vi "Refresh Param Channels.vi"(8 "error in (no error)":errorcluster, 10 "Label":T1, 11 "Param Ref in":T5 format="%.0x") -> (0 "error out":errorcluster, 3 "Param Ref out":T5 format="%.0x")   [LabVIEW 2015, in "AIT 429 System Explorer.lvlib"]
uses:
  AIT 429 System Explorer.lvlib
  <vilib>/NI Veristand/Custom Device API/Custom Device Item Ref.ctl
  Controls/AIT_Label.ctl
  Controls/AIT_Word.ctl
  Controls/ARINCParam.ctl
  Shared/Controls and Global/TransferType.ctl
  <vilib>/NI Veristand/Custom Device API/Custom Device Channel Type.ctl
  Shared/Controls and Global/Global.vi
  <vilib>/NI Veristand/Custom Device API/Set Item Property (Variant).vi
  <vilib>/NI Veristand/Custom Device Tools/Custom Device Utility Library/NI VeriStand - Search for All Items by GUID.vi
  Shared/AIT 429 Shared.lvlib
  <vilib>/NI Veristand/Custom Device Tools/Custom Device Utility Library/Custom Device Utility Library.lvlib
  <vilib>/NI Veristand/Custom Device API/Custom Device API.lvlib
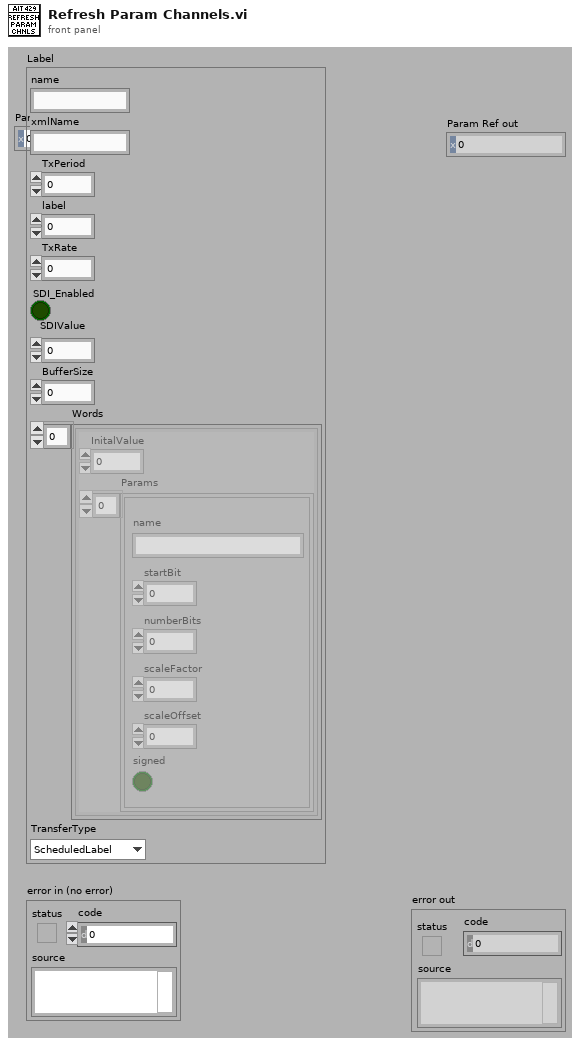
[diagram p1: front panel]
types:
  T1 = typedef "AIT 429 System Explorer.lvlib/AIT_Label.ctl" = cluster{"name":string, "xmlName":string, "TxPeriod":u32, "label":u32, "TxRate":dbl, "SDI_Enabled":bool, "SDIValue":u8, "BufferSize":u32, "Words":T2[], "TransferType":T4}
  T2 = typedef "AIT 429 System Explorer.lvlib/AIT_Word.ctl" = cluster{"InitalValue":u32, "Params":T3[]}
  T3 = typedef "AIT 429 System Explorer.lvlib/ARINCParam.ctl" = cluster{"name":string, "startBit":i32, "numberBits":i32, "scaleFactor":dbl, "scaleOffset":dbl, "signed":bool}
  T4 = typedef "AIT 429 Shared.lvlib/TransferType.ctl" = enum16{"ScheduledLabel", "Acyclic", "Block", "Strobe"}
  T5 = typedef "Custom Device API.lvlib/Custom Device Item Ref.ctl" = u64
  T6 = typedef "Custom Device API.lvlib/Custom Device Channel Type.ctl" = enum16{"Input", "Output"}
  T7 = typedef "Custom Device API.lvlib/Custom Device Item Info.ctl" = cluster{"Name":string, "Is Channel":bool, "GUID":string, "Is Waveform":bool}
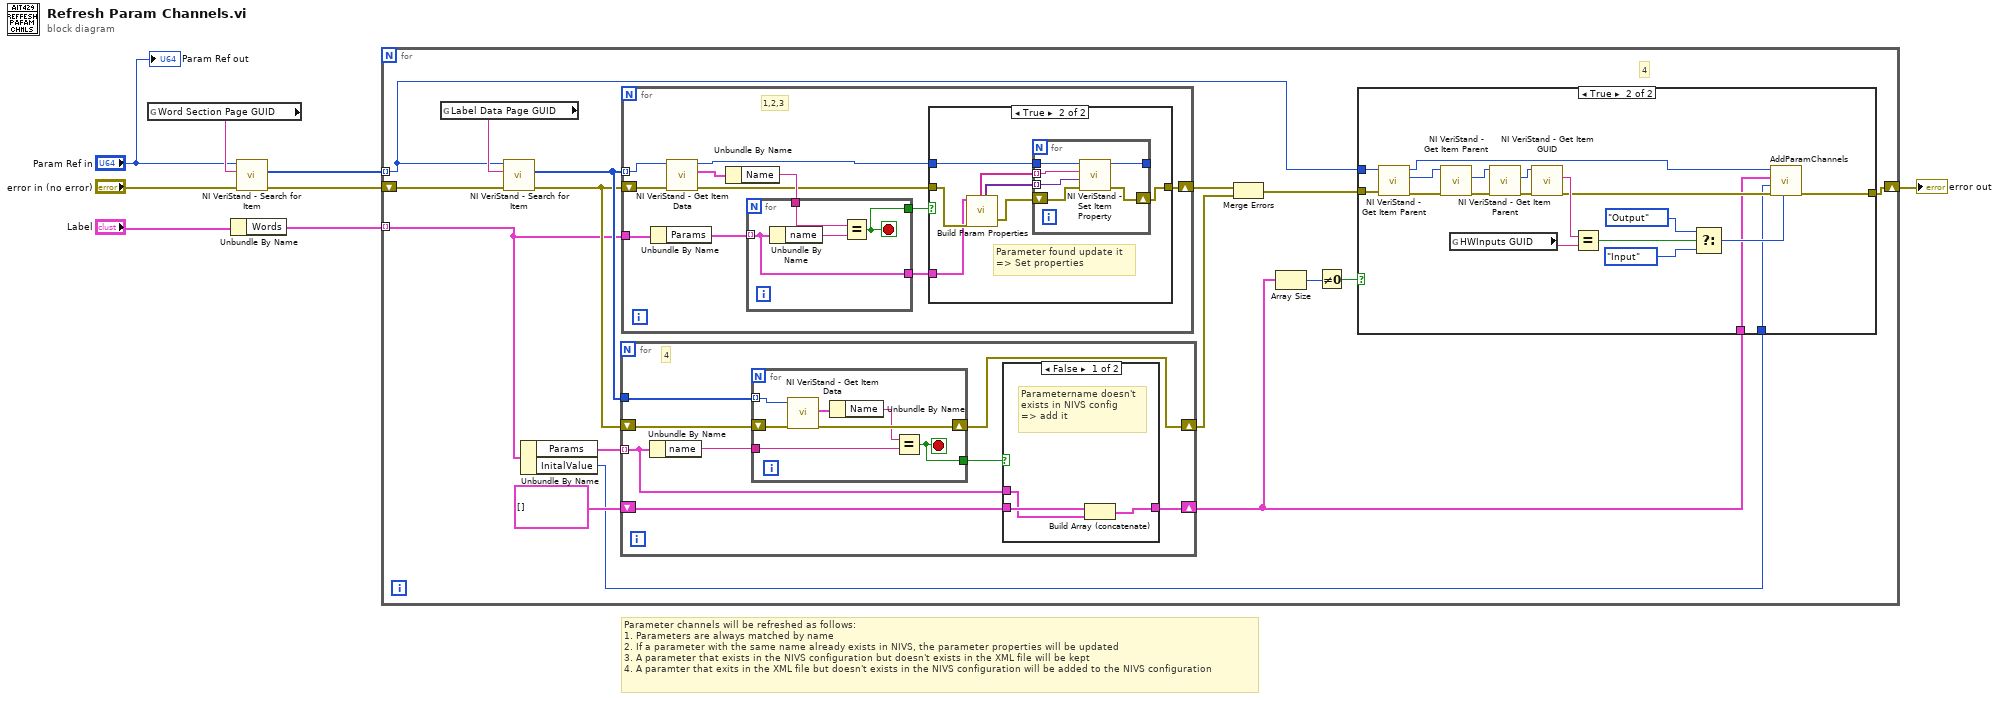
[diagram p0: block diagram]
diagram:
  # "Parameter channels will be refreshed as follows:\n1. Parameters are always matched by name\n2. If a parameter with the same name already exists in NIVS, the parameter properties will be updated\n3. A parameter that exists in the NIVS configuration but doesn't exists in the XML file will be kept\n4. A paramter that exits in the XML file but doesn't exists in the NIVS configuration will be added to the NIVS configuration"
  n1 = global read "Global.vi" "Word Section Page GUID"() -> (w6:string)
  n2 = Unbundle By Name("Label") -> ("Words"=w4:T2[])
  n3 = call-poly <vilib>:"NI VeriStand - Search for Item.vi"("error in"="error in (no error)", "Item GUID"=w6, "Section Ref in"="Param Ref in") -> ("error out"=w2:errorcluster, "Item Refs"=w5:T5[])  [unwired: 5 in, 2 out]
  n4 = for {
    tunnel: w5 -> [w9] mode=indexing
    tunnel: w4 -> [w11] mode=indexing
    shift-right: [w13] -> w7
    shift-left: w2 -> [w10]
    # "4"
    n5 = global read "Global.vi" "Label Data Page GUID"() -> (w24:string)
    n6 = call-poly <vilib>:"NI VeriStand - Search for Item.vi"("error in"=w10, "Item GUID"=w24, "Section Ref in"=w9) -> ("error out"=w21:errorcluster, "Item Refs"=w22:T5[])  [unwired: 5 in, 2 out]
    n7 = Unbundle By Name(w11) -> ("Params"=w23:T3[], "InitalValue"=w12:u32)
    n8 = for {
      tunnel: w23 -> [w46] mode=indexing
      tunnel: w22 -> [w52]
      shift-right: [w47] -> w14
      shift-left: T3[] [] ("Params") -> [w48]
      shift-right: [w45] -> w19
      shift-left: w21 -> [w51]
      # "4"
      n9 = Unbundle By Name(w46) -> ("name"=w50:string)
      n10 = for {
        tunnel: w52 -> [w62] mode=indexing
        shift-right: [w60] -> w45
        shift-left: w51 -> [w63]
        tunnel: w50 -> [w59]
        tunnel: [w57] -> w49
        stop <- w57 stop-if-true
        n11 = call <vilib>:"NI VeriStand - Get Item Data.vi"("error in (no error)"=w63, "Item Ref in"=w62) -> ("error out"=w60:errorcluster, "Item Info"=w61:T7)  [unwired: 6 in, 2 out]
        n12 = Unbundle By Name(w61) -> ("Name"=w58:string)
        n13 = Equal?(x=w58, y=w59) -> (x = y?=w57:bool)
      }
      n14 = case shown="False" w49 {
        tunnel: w48 -> [w55 w56]
        tunnel: [w54 w56] -> w47
        tunnel: w46 -> [w53 _]
        frame False {
          # "Parametername doesn't\nexists in NIVS config\n=> add it"
          n15 = Build Array (concatenate)(w55, w53) -> (w54:T3[])
        }
        frame True {
          # "Parametername \nexists in both NIVS\nconfiguration and\nXML file\n=> Nothing to do"
        }
      }
    }
    n16 = for {
      shift-right: [w64] -> w18
      shift-left: w21 -> [w71]
      tunnel: w22 -> [w72] mode=indexing
      tunnel: w11 -> [w74]
      # "1,2,3"
      n17 = Unbundle By Name(w74) -> ("Params"=w73:T3[])
      n18 = call <vilib>:"NI VeriStand - Get Item Data.vi"("error in (no error)"=w71, "Item Ref in"=w72) -> ("error out"=w66:errorcluster, "Item Info"=w70:T7, "Item Ref out"=w67:T5)  [unwired: 6 in, 1 out]
      n19 = Unbundle By Name(w70) -> ("Name"=w69:string)
      n20 = for {
        tunnel: w73 -> [w89] mode=indexing
        tunnel: w69 -> [w91]
        tunnel: [w90] -> w68
        tunnel: [w89] -> w65
        stop <- w90 stop-if-true
        n21 = Unbundle By Name(w89) -> ("name"=w92:string)
        n22 = Equal?(x=w91, y=w92) -> (x = y?=w90:bool)
      }
      n23 = case shown="True" w68 {
        tunnel: w67 -> [_ w79]
        tunnel: w66 -> [w75 w82]
        tunnel: w65 -> [_ w81]
        tunnel: [w75 w76] -> w64
        frame False {
          # "Parameter not in XML\nDo not change it"
        }
        frame True {
          # "Parameter found update it\n=> Set properties"
          n24 = call "Build Param Properties.vi"("ARINC Parameter"=w81, "error in (no error)"=w82) -> ("Prop Names"=w77:string[], "Prop Values"=w78:variant[], "error out"=w80:errorcluster)  [unwired: 9 in, 6 out]
          n25 = for {
            shift-right: [w87] -> w76
            shift-left: w80 -> [w88]
            tunnel: [w86] -> _
            tunnel: w79 -> [w85]
            tunnel: w78 -> [w84] mode=indexing
            tunnel: w77 -> [w83] mode=indexing
            n26 = call-poly <vilib>:"NI VeriStand - Set Item Property.vi"("error in (no error)"=w88, "Value"=w84, "Property Name"=w83, "Item Ref in"=w85) -> ("error out"=w87:errorcluster, "Item Ref out"=w86:T5)  [unwired: 5 in, 1 out]
          }
        }
      }
    }
    n27 = Merge Errors(w18, w19) -> (w15:errorcluster)
    n28 = Array Size(array=w14) -> (size(s)=w17:i32)
    n29 = Not Equal To 0?(x=w17) -> (x != 0?=w16:bool)
    n30 = case shown="True" w16 {
      tunnel: w15 -> [w25 w29]
      tunnel: w12 -> [_ w33]
      tunnel: w14 -> [_ w32]
      tunnel: [w25 w31] -> w13
      tunnel: w9 -> [_ w26]
      frame False {
      }
      frame True {
        n31 = call <vilib>:"NI VeriStand - Get Item Parent.vi"("error in (no error)"=w29, "Item Ref in"=w26) -> ("error out"=w30:errorcluster, "Parent Ref"=w28:T5, "Item Ref out"=w27:T5)  [unwired: 6 in, 1 out]
        n32 = call <vilib>:"NI VeriStand - Get Item Parent.vi"("error in (no error)"=w30, "Item Ref in"=w28) -> ("error out"=w36:errorcluster, "Parent Ref"=w39:T5)  [unwired: 6 in, 2 out]
        n33 = global read "Global.vi" "HWInputs GUID"() -> (w42:string)
        n34 = call <vilib>:"NI VeriStand - Get Item Parent.vi"("error in (no error)"=w36, "Item Ref in"=w39) -> ("error out"=w37:errorcluster, "Parent Ref"=w38:T5)  [unwired: 6 in, 2 out]
        n35 = call <vilib>:"NI VeriStand - Get Item GUID.vi"("error in (no error)"=w37, "Item Ref in"=w38) -> ("error out"=w35:errorcluster, "GUID"=w43:string)  [unwired: 7 in, 1 out]
        n36 = Equal?(x=w43, y=w42) -> (x = y?=w44:bool)
        n37 = Select(t=Custom_Device_Channel_Type."Output" ("Type"), s=w44, f=Custom_Device_Channel_Type."Input" ("Type")) -> (s? t:f=w34:T6)
        n38 = call "AddParamChannels.vi"("Type"=w34, "error in"=w35, "Initial Value"=w33, "Parameters to add"=w32, "Node Ref In"=w27) -> ("error out"=w31:errorcluster)  [unwired: 5 in, 1 out]
      }
    }
  }
  "error out" <- w7
  "Param Ref out" <- "Param Ref in"
